vi "toml_read_string.vi"(7 "section":string[](array[string]), 8 "error in (no error)":errorcluster, 9 "default":string, 10 "key":string[](array[string]), 11 "path in":path) -> (0 "error out":errorcluster, 1 "value":string, 2 "exists?":bool, 3 "path out":path)   [LabVIEW 2017]
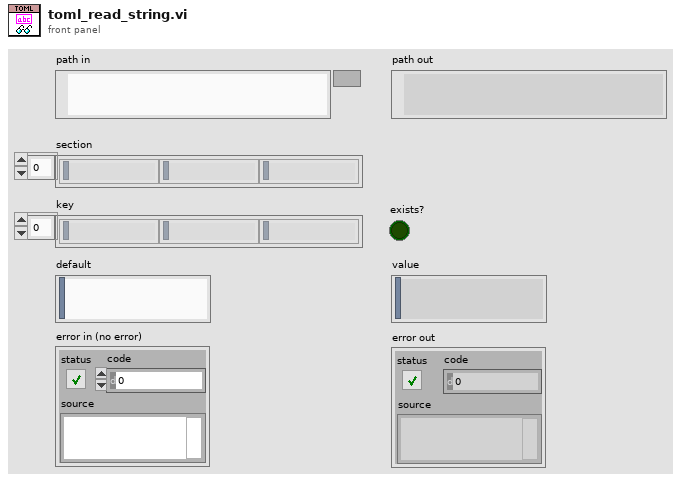
[diagram p1: front panel]
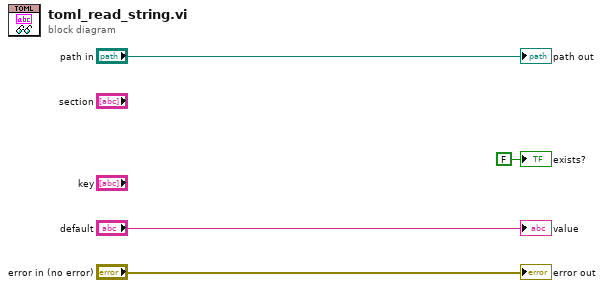
[diagram p0: block diagram]
diagram:
  "error out" <- "error in (no error)"
  "value" <- "default"
  "exists?" <- FALSE ("exists?")
  "path out" <- "path in"
